vi "writeToTiff.vi"(3 "error in":errorcluster, 4 "Save progress":refnum<vi>, 5 "Updated camera":T2, 6 "File Ctrl":T3={"Subject ID"="", "Eye"=FALSE, "Output Path"=path "E:/", "String"="OS", "String 2"="OD"}) -> (0 "error out":errorcluster)   [LabVIEW 2017]
uses:
  <vilib>/vision/Image Controls.llb/IMAQ Image.ctl
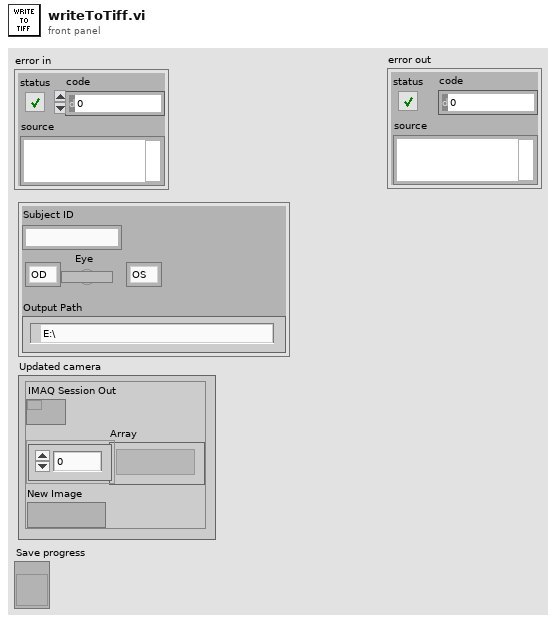
[diagram p1: front panel]
types:
  T1 = typedef "IMAQ Image.ctl" = refnum<image>
  T2 = cluster{"IMAQ Session Out":refnum<k11>, "Array":T1[], "New Image":T1}
  T3 = cluster{"Subject ID":string, "Eye":bool, "Output Path":path, "String":string, "String 2":string}
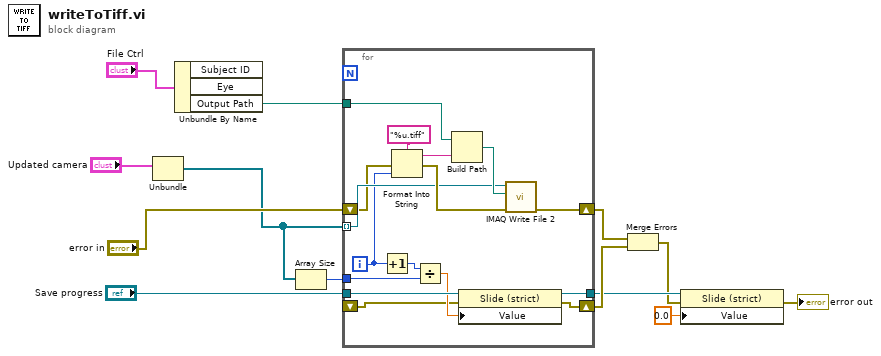
[diagram p0: block diagram]
diagram:
  n1 = Unbundle("Updated camera") -> ("Array"=w9:T1[])  [unwired: 2 out]
  n2 = Unbundle By Name("File Ctrl") -> ("Output Path"=w12:path)  [unwired: 2 out]
  n3 = Array Size(array=w9) -> (size(s)=w8:i32)
  n4 = for {
    tunnel: w12 -> [w25]
    tunnel: w9 -> [w24] mode=indexing
    shift-right: [w22] -> w5
    shift-left: "error in" -> [w23]
    tunnel: w8 -> [w19]
    tunnel: "Save progress" -> [w18]
    shift-right: [w16] -> w6
    shift-left: _ -> [w15]
    tunnel: [w14] -> w4
    i -> [w21]
    n5 = Increment(x=w21) -> (x+1=w20:i32)
    n6 = Format Into String(format string="%u.tiff" ("string"), error in=w23, w21) -> (resulting string=w26:string, error out=w28:errorcluster)  [unwired: 1 in]
    n7 = Divide(x=w20, y=w19) -> (x/y=w17:dbl)
    n8 = Build Path(base path=w25, name or relative path=w26) -> (appended path=w29:path)
    n9 = property class="Slide (strict)"(reference=w18, error in=w15, "Value"=w17) -> (reference out=w14:refnum<vi>, error out=w16:errorcluster)
    n10 = call-poly "IMAQ Write File 2"("error in (no error)"=w28, "File Path"=w29, "Image"=w24) -> ("error out"=w22:errorcluster)  [unwired: 7 in, 1 out]
  }
  n11 = Merge Errors(w5, w6) -> (w2:errorcluster)
  n12 = property class="Slide (strict)"(reference=w4, error in=w2, "Value"=sgl 0.0) -> (error out=→"error out":errorcluster)  [unwired: 1 out]
